vi "Write Thermo Channel.vi"(8 "error in (no error)":errorcluster, 10 "Thermo Channel Setting":T1={"Numeric"=0.5, "Combo"="", "String"="", "Boolean"=FALSE} {"Numeric" format="%#_f"}, 11 "Thermo Channel configuration in":refnum<class "Thermo Channel configuration.lvclass">) -> (0 "error out":errorcluster, 3 "Thermo Channel configuration out":refnum<class "Thermo Channel configuration.lvclass">)   [LabVIEW 2025, in "Thermo.lvlib" / "Thermo Channel configuration.lvclass"]
uses:
  Thermo Channel configuration.lvclass
  Thermo Channel configuration.lvclass/Thermo Channel configuration.ctl
  Channel Setting.ctl
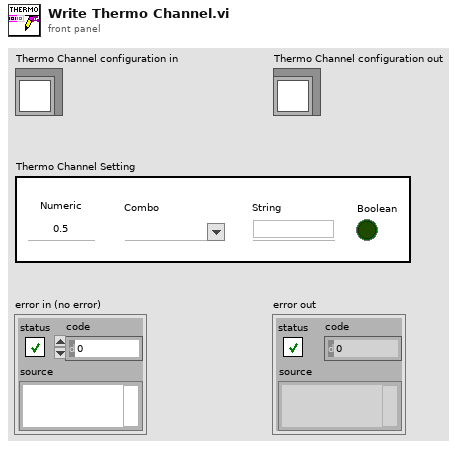
[diagram p1: front panel]
types:
  T1 = typedef "Thermo.lvlib/Thermo Channel configuration.lvclass/Channel Setting.ctl" = cluster{"Numeric":dbl, "Combo":string, "String":string, "Boolean":bool}
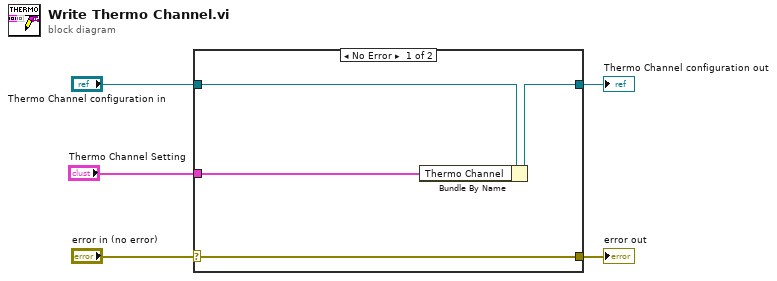
[diagram p0: block diagram]
diagram:
  n1 = case shown="No Error" "error in (no error)" {
    selector: "error in (no error)" -> [w9 w10]
    tunnel: [w9 w10] -> w4
    tunnel: [w7 w11] -> w2
    tunnel: "Thermo Channel configuration in" -> [w8 w11]
    tunnel: "Thermo Channel Setting" -> [w6 _]
    frame No Error {
      n2 = Bundle By Name(cluster=w8, "Thermo Channel"=w6) -> (w7:refnum<class "Thermo Channel configuration.lvclass">)
    }
    frame Error {
    }
  }
  "error out" <- w4
  "Thermo Channel configuration out" <- w2
